vi "kethley_INI_24xx.vi"(9 "Function (0: Volts) in":u16(ring) items=["Volts", "Current", "Resistance"], 10 "Source Compaliance":dbl, 11 "VISA Return in":refnum<visa-resource-name>) -> (1 "VISA resource name out":refnum<visa-resource-name>)   [LabVIEW 2020]
uses:
  <instrlib>/Keithley 24XX/Keithley 24XX.lvlib
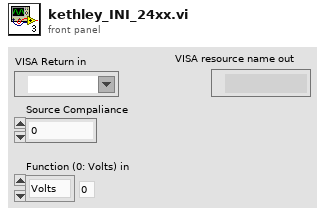
[diagram p1: front panel]
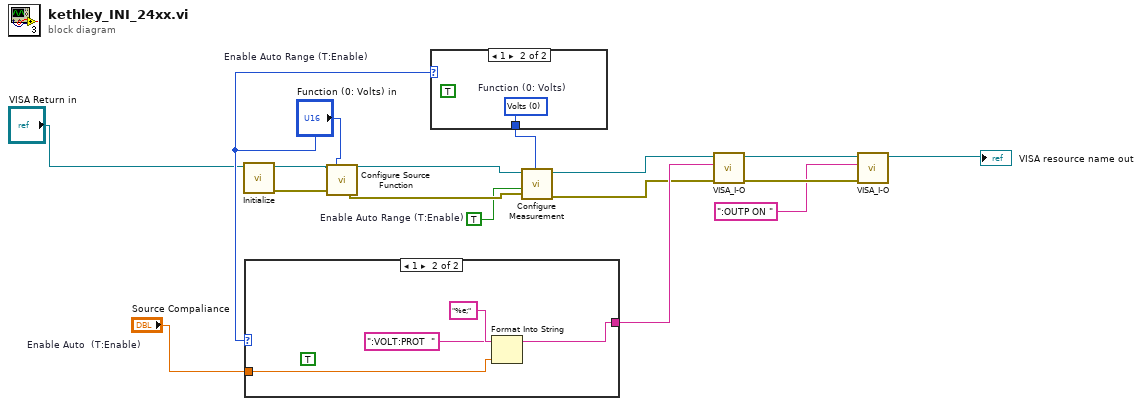
[diagram p0: block diagram]
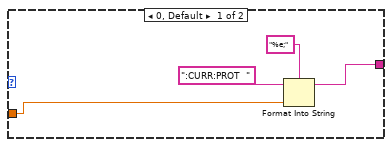
[diagram p2: hidden frame]
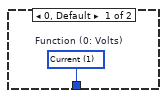
[diagram p3: hidden frame]
diagram:
  (unwired) TRUE  # Enable Auto  (T:Enable)
  w8 = TRUE  # Enable Auto Range (T:Enable)
  (unwired) TRUE  # Enable Auto Range (T:Enable)
  n1 = call <instrlib>:"Initialize.vi"("VISA resource name"="VISA Return in") -> ("error out"=w10:errorcluster, "VISA resource name out"=w6:refnum<visa-resource-name>)  [unwired: 9 in]
  n2 = case shown="1" "Function (0: Volts) in" {
    tunnel: [w17 w22] -> w14
    tunnel: "Source Compaliance" -> [w20 w21]
    frame 0, Default {
      n3 = Format Into String(format string="%e;", initial string=":CURR:PROT  " ("write buffer (\"\")"), w20) -> (resulting string=w17:string)  [unwired: 1 in, 1 out]
    }
    frame 1 {
      n4 = Format Into String(format string="%e;", initial string=":VOLT:PROT  " ("write buffer (\"\")"), w21) -> (resulting string=w22:string)  [unwired: 1 in, 1 out]
    }
  }
  n5 = call <instrlib>:"Configure Source Function.vi"("VISA resource name"=w6, "Function  (0: Voltage)"="Function (0: Volts) in", "error in (no error)"=w10) -> ("VISA resource name out"=w13:refnum<visa-resource-name>, "error out"=w12:errorcluster)  [unwired: 11 in]
  n6 = case shown="1" "Function (0: Volts) in" {
    tunnel: [w25 w26] -> w7
    frame 0, Default {
      w25 = u16 1 items=["Volts", "Current", "Resistance"]  # Function (0: Volts)
    }
    frame 1 {
      w26 = u16 0 items=["Volts", "Current", "Resistance"]  # Function (0: Volts)
    }
  }
  n7 = call <instrlib>:"Configure Measurement.vi"("error in (no error)"=w12, "Enable Auto Range (T:Enable)"=w8, "Function (0: Volts)"=w7, "VISA resource name"=w13) -> ("error out"=w11:errorcluster, "VISA resource name out"=w9:refnum<visa-resource-name>)  [unwired: 6 in]
  n8 = call "VISA_I-O.vi"("error in (no error)"=w11, "write buffer"=w14, "VISA resource name"=w9) -> ("error out"=w2:errorcluster, "VISA resource name out"=w4:refnum<visa-resource-name>)  [unwired: 6 in, 1 out]
  n9 = call "VISA_I-O.vi"("error in (no error)"=w2, "write buffer"=":OUTP ON " ("write buffer (\"\")"), "VISA resource name"=w4) -> ("VISA resource name out"=→"VISA resource name out":refnum<visa-resource-name>)  [unwired: 6 in, 2 out]
